vi "BinanceAPI_hmacSHA256.vi"(7 "Key":string, 8 "error In":errorcluster, 11 "String to Encode":string) -> (0 "error Out":errorcluster, 3 "Hash String":string)   [LabVIEW 2022 SP3]
doc: "Calculates the SHA256 HMAC signature"
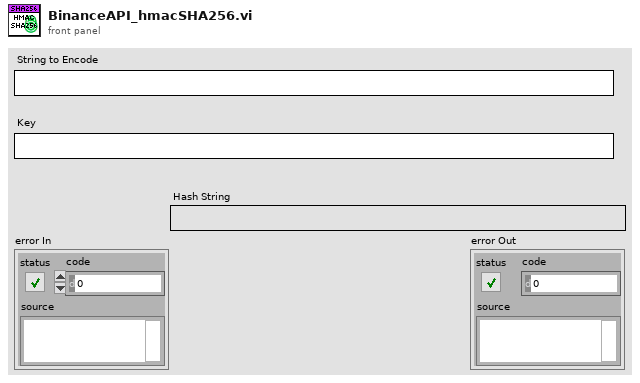
[diagram p1: front panel]
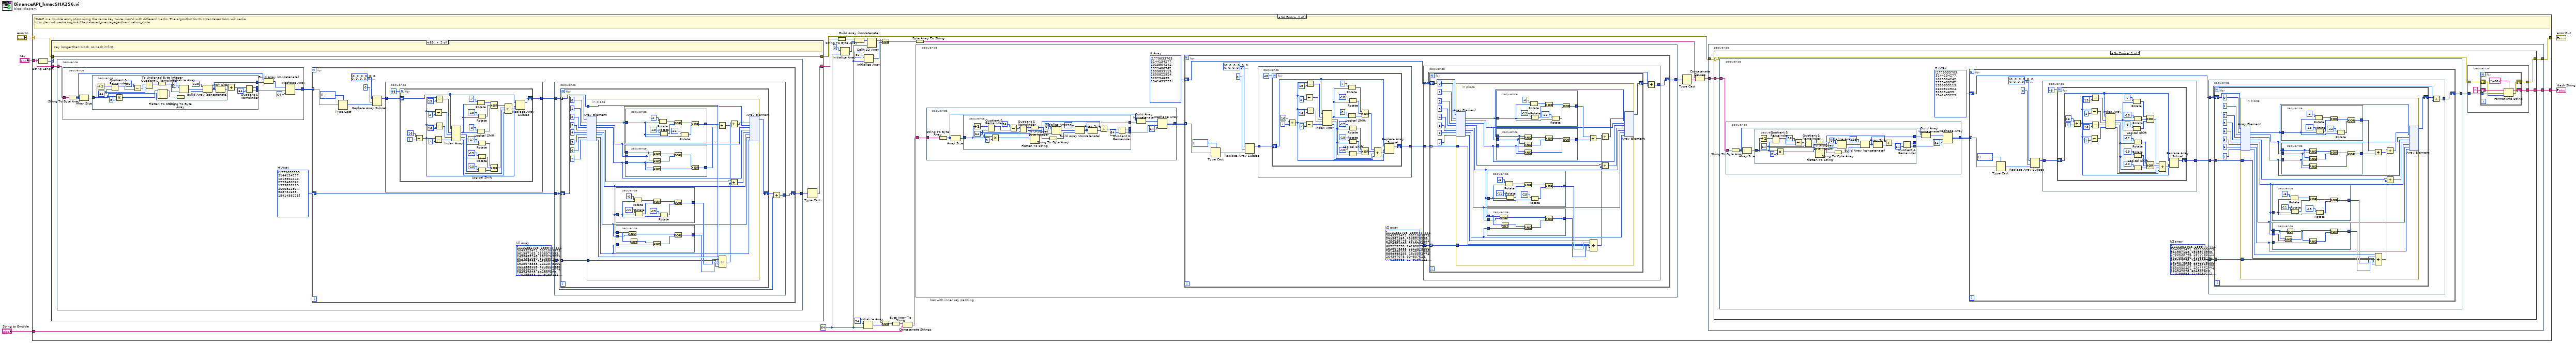
[diagram p0: block diagram]
diagram:
  n1 = case shown="No Error" "error In" {
    selector: "error In" -> [w29 w497]
    tunnel: "Key" -> [w30 _]
    tunnel: "String to Encode" -> [w16 _]
    tunnel: [w13 w497] -> w2
    tunnel: [w12 _] -> w1
    frame No Error {
      w9 = 64 ("dimension size")
      # "has with inner key padding"
      # "HMAC is a double encryption uisng the same key twice, xorr'd with different masks. The algorithm for this was taken from wikipedia \nhttps://en.wikipedia.org/wiki/Hash-based_message_authentication_code"
      n2 = String Length(string=w30) -> (length=w31:i32)
      n3 = case shown="65.." w31 {
        tunnel: w30 -> [w346 w350]
        tunnel: w29 -> [w345 w349]
        tunnel: [w345 w349] -> w11
        tunnel: [w346 w348] -> w28
        frame 0, Default {
        }
        frame 65.. {
          # "Key longer than block, so hash it first."
          n4 = stacked-sequence {
            tunnel: [w353] -> w347
            tunnel: w350 -> [w354]
            frame #0 {
              w351 = u32[] [1779033703, 3144134277, 1013904242, 2773480762, 1359893119, 2600822924, 528734635, 1541459225]  # H Array
              n5 = stacked-sequence {
                tunnel: [w358] -> w352
                tunnel: w354 -> [w355]
                frame #0 {
                  n6 = String To Byte Array(string=w355) -> (unsigned byte array=w359:u8[])
                  n7 = Array Size(array=w359) -> (size(s)=w361:i32)
                  n8 = stacked-sequence {
                    tunnel: [w363] -> _
                    tunnel: [w370] -> w356
                    tunnel: [w365] -> w360
                    tunnel: w361 -> [w379]
                    frame #0 {
                      w368 = i64 64 ("y")
                      n9 = Increment(x=w379) -> (x+1=w378:i32)
                      n10 = Quotient & Remainder(x=w378, y=w368) -> (x-y*floor(x/y)=w377:i64)  [unwired: 1 out]
                      n11 = Multiply(x=w379, y=i64 8) -> (x*y=w383:i64)
                      n12 = Subtract(x=i64 56, y=w377) -> (x-y=w369:i64)
                      n13 = Quotient & Remainder(x=w369, y=w368) -> (x-y*floor(x/y)=w366:i64)  [unwired: 1 out]
                      n14 = To Unsigned Byte Integer(number=w366) -> (unsigned 8bit integer=w380:u8)
                      n15 = Flatten To String(anything=w383) -> (data string=w381:string)  [unwired: 3 in, 2 out]
                      n16 = String To Byte Array(string=w381) -> (unsigned byte array=w382:u8[])
                      n17 = Initialize Array(u8 0, w380) -> (w374:u8[])
                      n18 = Build Array (concatenate)(u8 128, w374, w382) -> (w365:u8[])
                      n19 = Array Size(array=w365) -> (size(s)=w372:i32)
                      n20 = Add(x=w379, y=w372) -> (x+y=w364:i32)
                      n21 = Quotient & Remainder(x=w364, y=u64 64) -> (x-y*floor(x/y)=w363:u64, floor(x/y)=w370:u64)
                    }
                  }
                  n22 = Build Array (concatenate)(w359, w360) -> (w362:u8[])
                  n23 = Reshape Array(w362, w356, 64 ("dimension size")) -> (w358:u8[][])
                }
              }
              n24 = for {
                tunnel: w352 -> [w393] mode=indexing
                shift-right: [w386] -> w353
                shift-left: w351 -> [w387]
                w385 = u32[] [1116352408, 1899447441, 3049323471, 3921009573, 961987163, 1508970993, 2453635748, 2870763221, 3624381080, 310598401, 607225278, 1426881987, 1925078388, 2162078206, 2614888103, 3248222580, 3835390401, 4022224774, 264347078, 604807628, 770255983, 1249150122, 1555081692, 1996064986, 2554220882, 2821834349, 2952996808, 3210313671, 3336571891, 3584528711, 113926993, 338241895, 666307205, 773529912, 1294757372, 1396182291, 1695183700, 1986661051, 2177026350, 2456956037, 2730485921, 2820302411, 3259730800, 3345764771, 3516065817, 3600352804, 4094571909, 275423344, 430227734, 506948616, 659060556, 883997877, 958139571, 1322822218, 1537002063, 1747873779, 1955562222, 2024104815, 2227730452, 2361852424, 2428436474, 2756734187, 3204031479, 3329325298]  # k[] array
                n25 = Type Cast(type=u32[] [], x=w393) -> (*(type *) &x=w391:u32[])
                n26 = Replace Array Subset(array=u32[] [0, 0, 0, 0, 0, 0, 0, 0, 0, 0, 0, 0, 0, 0, 0, 0, 0, 0, 0, 0, 0, 0, 0, 0, 0, 0, 0, 0, 0, 0, 0, 0, 0, 0, 0, 0, 0, 0, 0, 0, 0, 0, 0, 0, 0, 0, 0, 0, 0, 0, 0, 0, 0, 0, 0, 0, 0, 0, 0, 0, 0, 0, 0, 0], new element=w391, index=0) -> (w389:u32[])
                n27 = stacked-sequence {
                  tunnel: [w462] -> w388
                  tunnel: w389 -> [w463]
                  frame #0 {
                    n28 = for {
                      N: 48 -> [_]
                      shift-right: [w467] -> w462
                      shift-left: w463 -> [w490]
                      i -> [w496]
                      n29 = Add(x=16, y=w496) -> (x+y=w465:i32)
                      n30 = Subtract(x=w465, y=2) -> (x-y=w492:i32)
                      n31 = Subtract(x=w465, y=7) -> (x-y=w486:i32)
                      n32 = Subtract(x=w465, y=15) -> (x-y=w494:i32)
                      n33 = Subtract(x=w465, y=16) -> (x-y=w489:i32)
                      n34 = Index Array(array=w490, index #1=w494, index #2=w492, index #3=w489, index #4=w486) -> (element #1=w483:u32, element #2=w476:u32, element #3=w469:u32, element #4=w468:u32)
                      n35 = Rotate(1:w483, 2:i16 -7 ("y")) -> (0:w481:u32)
                      n36 = Logical Shift(y=i16 -3, x=w483) -> (x << y=w479:u32)
                      n37 = Rotate(1:w483, 2:i16 -18 ("y")) -> (0:w480:u32)
                      n38 = Rotate(1:w476, 2:i16 -17 ("y")) -> (0:w472:u32)
                      n39 = Rotate(1:w476, 2:i16 -19 ("y")) -> (0:w473:u32)
                      n40 = Logical Shift(y=i16 -10, x=w476) -> (x << y=w474:u32)
                      n41 = Compound Arithmetic op=XOR(w481, w480, w479) -> (w471:u32)
                      n42 = Compound Arithmetic op=XOR(w472, w473, w474) -> (w470:u32)
                      n43 = Compound Arithmetic op=ADD(w471, w470, w469, w468) -> (w466:u32)
                      n44 = Replace Array Subset(array=w490, new element=w466, index=w465) -> (w467:u32[])
                    }
                  }
                }
                n45 = stacked-sequence {
                  tunnel: [w398] -> w386
                  tunnel: w385 -> [w394]
                  tunnel: w387 -> [w396]
                  tunnel: w388 -> [w395]
                  frame #0 {
                    n46 = for {
                      tunnel: w395 -> [w401] mode=indexing
                      tunnel: w394 -> [w400] mode=indexing
                      shift-right: [w399] -> w397
                      shift-left: w396 -> [w410]
                      n47 = in-place {
                        in-place-border: w401 -> [w425]
                        in-place-border: w400 -> [w424]
                        n48 = in-place-array #1(w410, 0, 1, 2, 3, 4, 5, 6, 7) -> (w414:u32, w415:u32, w416:u32, w418:u32, w419:u32, w420:u32, w421:u32, w428:u32)
                        n49 = stacked-sequence {
                          tunnel: [w444] -> w427
                          tunnel: w419 -> [w439]
                          frame #0 {
                            n50 = Rotate(1:w439, 2:i16 -6 ("y")) -> (0:w440:u32)
                            n51 = Rotate(1:w439, 2:i16 -11 ("y")) -> (0:w441:u32)
                            n52 = Exclusive Or(1:w441, 2:w440) -> (0:w442:u32)
                            n53 = Rotate(1:w439, 2:i16 -25 ("y")) -> (0:w443:u32)
                            n54 = Exclusive Or(1:w443, 2:w442) -> (0:w444:u32)
                          }
                        }
                        n55 = stacked-sequence {
                          tunnel: [w435] -> w426
                          tunnel: w421 -> [w432]
                          tunnel: w420 -> [w429]
                          tunnel: w419 -> [w430]
                          frame #0 {
                            n56 = And(x=w430, y=w429) -> (x .and. y?=w433:u32)
                            n57 = Not(x=w430) -> (.not. x?=w431:u32)
                            n58 = And(x=w431, y=w432) -> (x .and. y?=w434:u32)
                            n59 = Exclusive Or(1:w434, 2:w433) -> (0:w435:u32)
                          }
                        }
                        n60 = stacked-sequence {
                          tunnel: [w461] -> w423
                          tunnel: w414 -> [w456]
                          frame #0 {
                            n61 = Rotate(1:w456, 2:i16 -2 ("y")) -> (0:w457:u32)
                            n62 = Rotate(1:w456, 2:i16 -13 ("y")) -> (0:w458:u32)
                            n63 = Exclusive Or(1:w458, 2:w457) -> (0:w459:u32)
                            n64 = Rotate(1:w456, 2:i16 -22 ("y")) -> (0:w460:u32)
                            n65 = Exclusive Or(1:w460, 2:w459) -> (0:w461:u32)
                          }
                        }
                        n66 = stacked-sequence {
                          tunnel: [w452] -> w422
                          tunnel: w416 -> [w446]
                          tunnel: w415 -> [w445]
                          tunnel: w414 -> [w447]
                          frame #0 {
                            n67 = And(x=w447, y=w445) -> (x .and. y?=w448:u32)
                            n68 = And(x=w447, y=w446) -> (x .and. y?=w449:u32)
                            n69 = And(x=w445, y=w446) -> (x .and. y?=w451:u32)
                            n70 = Exclusive Or(1:w449, 2:w448) -> (0:w450:u32)
                            n71 = Exclusive Or(1:w451, 2:w450) -> (0:w452:u32)
                          }
                        }
                        n72 = Add(x=w423, y=w422) -> (x+y=w412:u32)
                        n73 = Compound Arithmetic op=ADD(w428, w427, w426, w425, w424) -> (w413:u32)
                        n74 = Add(x=w413, y=w412) -> (x+y=w411:u32)
                        n75 = Add(x=w418, y=w413) -> (x+y=w417:u32)
                        n76 = in-place-array #1(w411, w414, w415, w416, w417, w419, w420, w421) -> (w399:u32[])  [unwired: 8 out]
                      }
                    }
                    n77 = Add(x=w397, y=w396) -> (x+y=w398:u32[])
                  }
                }
              }
            }
          }
          n78 = Type Cast(x=w347) -> (*(type *) &x=w348:string)  [unwired: 1 in]
        }
      }
      n79 = String To Byte Array(string=w28) -> (unsigned byte array=w27:u8[])
      n80 = Initialize Array(u8 0 ("element"), w9) -> (w25:u8[])
      n81 = Build Array (concatenate)(w27, w25) -> (w24:u8[])
      n82 = Initialize Array(u8 54, w9) -> (w20:u8[])
      n83 = Initialize Array(u8 92, w9) -> (w21:u8[])
      n84 = Split 1D Array(array=w24, index=w9) -> (first subarray=w19:u8[])  [unwired: 1 out]
      n85 = Exclusive Or(1:w21, 2:w19) -> (0:w18:u8[])
      n86 = Exclusive Or(1:w20, 2:w19) -> (0:w17:u8[])
      n87 = Byte Array To String(unsigned byte array=w17) -> (string=w10:string)
      n88 = Concatenate Strings(w10, w16) -> (w8:string)
      n89 = Byte Array To String(unsigned byte array=w18) -> (string=w15:string)
      n90 = stacked-sequence {
        tunnel: [w201] -> w7
        tunnel: w8 -> [w202]
        frame #0 {
          w199 = u32[] [1779033703, 3144134277, 1013904242, 2773480762, 1359893119, 2600822924, 528734635, 1541459225]  # H Array
          n91 = stacked-sequence {
            tunnel: [w206] -> w200
            tunnel: w202 -> [w203]
            frame #0 {
              n92 = String To Byte Array(string=w203) -> (unsigned byte array=w207:u8[])
              n93 = Array Size(array=w207) -> (size(s)=w209:i32)
              n94 = stacked-sequence {
                tunnel: [w211] -> _
                tunnel: [w218] -> w204
                tunnel: [w213] -> w208
                tunnel: w209 -> [w227]
                frame #0 {
                  w216 = i64 64 ("y")
                  n95 = Increment(x=w227) -> (x+1=w226:i32)
                  n96 = Quotient & Remainder(x=w226, y=w216) -> (x-y*floor(x/y)=w225:i64)  [unwired: 1 out]
                  n97 = Multiply(x=w227, y=i64 8) -> (x*y=w231:i64)
                  n98 = Subtract(x=i64 56, y=w225) -> (x-y=w217:i64)
                  n99 = Quotient & Remainder(x=w217, y=w216) -> (x-y*floor(x/y)=w214:i64)  [unwired: 1 out]
                  n100 = To Unsigned Byte Integer(number=w214) -> (unsigned 8bit integer=w228:u8)
                  n101 = Flatten To String(anything=w231) -> (data string=w229:string)  [unwired: 3 in, 2 out]
                  n102 = String To Byte Array(string=w229) -> (unsigned byte array=w230:u8[])
                  n103 = Initialize Array(u8 0, w228) -> (w222:u8[])
                  n104 = Build Array (concatenate)(u8 128, w222, w230) -> (w213:u8[])
                  n105 = Array Size(array=w213) -> (size(s)=w220:i32)
                  n106 = Add(x=w227, y=w220) -> (x+y=w212:i32)
                  n107 = Quotient & Remainder(x=w212, y=u64 64) -> (x-y*floor(x/y)=w211:u64, floor(x/y)=w218:u64)
                }
              }
              n108 = Build Array (concatenate)(w207, w208) -> (w210:u8[])
              n109 = Reshape Array(w210, w204, 64 ("dimension size")) -> (w206:u8[][])
            }
          }
          n110 = for {
            tunnel: w200 -> [w241] mode=indexing
            shift-right: [w234] -> w201
            shift-left: w199 -> [w235]
            w233 = u32[] [1116352408, 1899447441, 3049323471, 3921009573, 961987163, 1508970993, 2453635748, 2870763221, 3624381080, 310598401, 607225278, 1426881987, 1925078388, 2162078206, 2614888103, 3248222580, 3835390401, 4022224774, 264347078, 604807628, 770255983, 1249150122, 1555081692, 1996064986, 2554220882, 2821834349, 2952996808, 3210313671, 3336571891, 3584528711, 113926993, 338241895, 666307205, 773529912, 1294757372, 1396182291, 1695183700, 1986661051, 2177026350, 2456956037, 2730485921, 2820302411, 3259730800, 3345764771, 3516065817, 3600352804, 4094571909, 275423344, 430227734, 506948616, 659060556, 883997877, 958139571, 1322822218, 1537002063, 1747873779, 1955562222, 2024104815, 2227730452, 2361852424, 2428436474, 2756734187, 3204031479, 3329325298]  # k[] array
            n111 = Type Cast(type=u32[] [], x=w241) -> (*(type *) &x=w239:u32[])
            n112 = Replace Array Subset(array=u32[] [0, 0, 0, 0, 0, 0, 0, 0, 0, 0, 0, 0, 0, 0, 0, 0, 0, 0, 0, 0, 0, 0, 0, 0, 0, 0, 0, 0, 0, 0, 0, 0, 0, 0, 0, 0, 0, 0, 0, 0, 0, 0, 0, 0, 0, 0, 0, 0, 0, 0, 0, 0, 0, 0, 0, 0, 0, 0, 0, 0, 0, 0, 0, 0], new element=w239, index=0) -> (w237:u32[])
            n113 = stacked-sequence {
              tunnel: [w310] -> w236
              tunnel: w237 -> [w311]
              frame #0 {
                n114 = for {
                  N: 48 -> [_]
                  shift-right: [w315] -> w310
                  shift-left: w311 -> [w338]
                  i -> [w344]
                  n115 = Add(x=16, y=w344) -> (x+y=w313:i32)
                  n116 = Subtract(x=w313, y=2) -> (x-y=w340:i32)
                  n117 = Subtract(x=w313, y=7) -> (x-y=w334:i32)
                  n118 = Subtract(x=w313, y=15) -> (x-y=w342:i32)
                  n119 = Subtract(x=w313, y=16) -> (x-y=w337:i32)
                  n120 = Index Array(array=w338, index #1=w342, index #2=w340, index #3=w337, index #4=w334) -> (element #1=w331:u32, element #2=w324:u32, element #3=w317:u32, element #4=w316:u32)
                  n121 = Rotate(1:w331, 2:i16 -7 ("y")) -> (0:w329:u32)
                  n122 = Logical Shift(y=i16 -3, x=w331) -> (x << y=w327:u32)
                  n123 = Rotate(1:w331, 2:i16 -18 ("y")) -> (0:w328:u32)
                  n124 = Rotate(1:w324, 2:i16 -17 ("y")) -> (0:w320:u32)
                  n125 = Rotate(1:w324, 2:i16 -19 ("y")) -> (0:w321:u32)
                  n126 = Logical Shift(y=i16 -10, x=w324) -> (x << y=w322:u32)
                  n127 = Compound Arithmetic op=XOR(w329, w328, w327) -> (w319:u32)
                  n128 = Compound Arithmetic op=XOR(w320, w321, w322) -> (w318:u32)
                  n129 = Compound Arithmetic op=ADD(w319, w318, w317, w316) -> (w314:u32)
                  n130 = Replace Array Subset(array=w338, new element=w314, index=w313) -> (w315:u32[])
                }
              }
            }
            n131 = stacked-sequence {
              tunnel: [w246] -> w234
              tunnel: w233 -> [w242]
              tunnel: w235 -> [w244]
              tunnel: w236 -> [w243]
              frame #0 {
                n132 = for {
                  tunnel: w243 -> [w249] mode=indexing
                  tunnel: w242 -> [w248] mode=indexing
                  shift-right: [w247] -> w245
                  shift-left: w244 -> [w258]
                  n133 = in-place {
                    in-place-border: w249 -> [w273]
                    in-place-border: w248 -> [w272]
                    n134 = in-place-array #2(w258, 0, 1, 2, 3, 4, 5, 6, 7) -> (w262:u32, w263:u32, w264:u32, w266:u32, w267:u32, w268:u32, w269:u32, w276:u32)
                    n135 = stacked-sequence {
                      tunnel: [w292] -> w275
                      tunnel: w267 -> [w287]
                      frame #0 {
                        n136 = Rotate(1:w287, 2:i16 -6 ("y")) -> (0:w288:u32)
                        n137 = Rotate(1:w287, 2:i16 -11 ("y")) -> (0:w289:u32)
                        n138 = Exclusive Or(1:w289, 2:w288) -> (0:w290:u32)
                        n139 = Rotate(1:w287, 2:i16 -25 ("y")) -> (0:w291:u32)
                        n140 = Exclusive Or(1:w291, 2:w290) -> (0:w292:u32)
                      }
                    }
                    n141 = stacked-sequence {
                      tunnel: [w283] -> w274
                      tunnel: w269 -> [w280]
                      tunnel: w268 -> [w277]
                      tunnel: w267 -> [w278]
                      frame #0 {
                        n142 = And(x=w278, y=w277) -> (x .and. y?=w281:u32)
                        n143 = Not(x=w278) -> (.not. x?=w279:u32)
                        n144 = And(x=w279, y=w280) -> (x .and. y?=w282:u32)
                        n145 = Exclusive Or(1:w282, 2:w281) -> (0:w283:u32)
                      }
                    }
                    n146 = stacked-sequence {
                      tunnel: [w309] -> w271
                      tunnel: w262 -> [w304]
                      frame #0 {
                        n147 = Rotate(1:w304, 2:i16 -2 ("y")) -> (0:w305:u32)
                        n148 = Rotate(1:w304, 2:i16 -13 ("y")) -> (0:w306:u32)
                        n149 = Exclusive Or(1:w306, 2:w305) -> (0:w307:u32)
                        n150 = Rotate(1:w304, 2:i16 -22 ("y")) -> (0:w308:u32)
                        n151 = Exclusive Or(1:w308, 2:w307) -> (0:w309:u32)
                      }
                    }
                    n152 = stacked-sequence {
                      tunnel: [w300] -> w270
                      tunnel: w264 -> [w294]
                      tunnel: w263 -> [w293]
                      tunnel: w262 -> [w295]
                      frame #0 {
                        n153 = And(x=w295, y=w293) -> (x .and. y?=w296:u32)
                        n154 = And(x=w295, y=w294) -> (x .and. y?=w297:u32)
                        n155 = And(x=w293, y=w294) -> (x .and. y?=w299:u32)
                        n156 = Exclusive Or(1:w297, 2:w296) -> (0:w298:u32)
                        n157 = Exclusive Or(1:w299, 2:w298) -> (0:w300:u32)
                      }
                    }
                    n158 = Add(x=w271, y=w270) -> (x+y=w260:u32)
                    n159 = Compound Arithmetic op=ADD(w276, w275, w274, w273, w272) -> (w261:u32)
                    n160 = Add(x=w261, y=w260) -> (x+y=w259:u32)
                    n161 = Add(x=w266, y=w261) -> (x+y=w265:u32)
                    n162 = in-place-array #2(w259, w262, w263, w264, w265, w267, w268, w269) -> (w247:u32[])  [unwired: 8 out]
                  }
                }
                n163 = Add(x=w245, y=w244) -> (x+y=w246:u32[])
              }
            }
          }
        }
      }
      n164 = Type Cast(x=w7) -> (*(type *) &x=w6:string)  [unwired: 1 in]
      n165 = Concatenate Strings(w15, w6) -> (w14:string)
      n166 = stacked-sequence {
        tunnel: [w34] -> w13
        tunnel: [w33] -> w12
        tunnel: w11 -> [w35]
        tunnel: w14 -> [w32]
        frame #0 {
          n167 = case shown="No Error" w35 {
            selector: w35 -> [w36 w198]
            tunnel: w32 -> [w40 _]
            tunnel: [w38 _] -> w33
            tunnel: [w37 w198] -> w34
            frame No Error {
              n168 = stacked-sequence {
                tunnel: [w54] -> w39
                tunnel: w40 -> [w55]
                frame #0 {
                  w52 = u32[] [1779033703, 3144134277, 1013904242, 2773480762, 1359893119, 2600822924, 528734635, 1541459225]  # H Array
                  n169 = stacked-sequence {
                    tunnel: [w59] -> w53
                    tunnel: w55 -> [w56]
                    frame #0 {
                      n170 = String To Byte Array(string=w56) -> (unsigned byte array=w60:u8[])
                      n171 = Array Size(array=w60) -> (size(s)=w62:i32)
                      n172 = stacked-sequence {
                        tunnel: [w64] -> _
                        tunnel: [w71] -> w57
                        tunnel: [w66] -> w61
                        tunnel: w62 -> [w80]
                        frame #0 {
                          w69 = i64 64 ("y")
                          n173 = Increment(x=w80) -> (x+1=w79:i32)
                          n174 = Quotient & Remainder(x=w79, y=w69) -> (x-y*floor(x/y)=w78:i64)  [unwired: 1 out]
                          n175 = Multiply(x=w80, y=i64 8) -> (x*y=w84:i64)
                          n176 = Subtract(x=i64 56, y=w78) -> (x-y=w70:i64)
                          n177 = Quotient & Remainder(x=w70, y=w69) -> (x-y*floor(x/y)=w67:i64)  [unwired: 1 out]
                          n178 = To Unsigned Byte Integer(number=w67) -> (unsigned 8bit integer=w81:u8)
                          n179 = Flatten To String(anything=w84) -> (data string=w82:string)  [unwired: 3 in, 2 out]
                          n180 = String To Byte Array(string=w82) -> (unsigned byte array=w83:u8[])
                          n181 = Initialize Array(u8 0, w81) -> (w75:u8[])
                          n182 = Build Array (concatenate)(u8 128, w75, w83) -> (w66:u8[])
                          n183 = Array Size(array=w66) -> (size(s)=w73:i32)
                          n184 = Add(x=w80, y=w73) -> (x+y=w65:i32)
                          n185 = Quotient & Remainder(x=w65, y=u64 64) -> (x-y*floor(x/y)=w64:u64, floor(x/y)=w71:u64)
                        }
                      }
                      n186 = Build Array (concatenate)(w60, w61) -> (w63:u8[])
                      n187 = Reshape Array(w63, w57, 64 ("dimension size")) -> (w59:u8[][])
                    }
                  }
                  n188 = for {
                    tunnel: w53 -> [w94] mode=indexing
                    shift-right: [w87] -> w54
                    shift-left: w52 -> [w88]
                    w86 = u32[] [1116352408, 1899447441, 3049323471, 3921009573, 961987163, 1508970993, 2453635748, 2870763221, 3624381080, 310598401, 607225278, 1426881987, 1925078388, 2162078206, 2614888103, 3248222580, 3835390401, 4022224774, 264347078, 604807628, 770255983, 1249150122, 1555081692, 1996064986, 2554220882, 2821834349, 2952996808, 3210313671, 3336571891, 3584528711, 113926993, 338241895, 666307205, 773529912, 1294757372, 1396182291, 1695183700, 1986661051, 2177026350, 2456956037, 2730485921, 2820302411, 3259730800, 3345764771, 3516065817, 3600352804, 4094571909, 275423344, 430227734, 506948616, 659060556, 883997877, 958139571, 1322822218, 1537002063, 1747873779, 1955562222, 2024104815, 2227730452, 2361852424, 2428436474, 2756734187, 3204031479, 3329325298]  # k[] array
                    n189 = Type Cast(type=u32[] [], x=w94) -> (*(type *) &x=w92:u32[])
                    n190 = Replace Array Subset(array=u32[] [0, 0, 0, 0, 0, 0, 0, 0, 0, 0, 0, 0, 0, 0, 0, 0, 0, 0, 0, 0, 0, 0, 0, 0, 0, 0, 0, 0, 0, 0, 0, 0, 0, 0, 0, 0, 0, 0, 0, 0, 0, 0, 0, 0, 0, 0, 0, 0, 0, 0, 0, 0, 0, 0, 0, 0, 0, 0, 0, 0, 0, 0, 0, 0], new element=w92, index=0) -> (w90:u32[])
                    n191 = stacked-sequence {
                      tunnel: [w163] -> w89
                      tunnel: w90 -> [w164]
                      frame #0 {
                        n192 = for {
                          N: 48 -> [_]
                          shift-right: [w168] -> w163
                          shift-left: w164 -> [w191]
                          i -> [w197]
                          n193 = Add(x=16, y=w197) -> (x+y=w166:i32)
                          n194 = Subtract(x=w166, y=2) -> (x-y=w193:i32)
                          n195 = Subtract(x=w166, y=7) -> (x-y=w187:i32)
                          n196 = Subtract(x=w166, y=15) -> (x-y=w195:i32)
                          n197 = Subtract(x=w166, y=16) -> (x-y=w190:i32)
                          n198 = Index Array(array=w191, index #1=w195, index #2=w193, index #3=w190, index #4=w187) -> (element #1=w184:u32, element #2=w177:u32, element #3=w170:u32, element #4=w169:u32)
                          n199 = Rotate(1:w184, 2:i16 -7 ("y")) -> (0:w182:u32)
                          n200 = Logical Shift(y=i16 -3, x=w184) -> (x << y=w180:u32)
                          n201 = Rotate(1:w184, 2:i16 -18 ("y")) -> (0:w181:u32)
                          n202 = Rotate(1:w177, 2:i16 -17 ("y")) -> (0:w173:u32)
                          n203 = Rotate(1:w177, 2:i16 -19 ("y")) -> (0:w174:u32)
                          n204 = Logical Shift(y=i16 -10, x=w177) -> (x << y=w175:u32)
                          n205 = Compound Arithmetic op=XOR(w182, w181, w180) -> (w172:u32)
                          n206 = Compound Arithmetic op=XOR(w173, w174, w175) -> (w171:u32)
                          n207 = Compound Arithmetic op=ADD(w172, w171, w170, w169) -> (w167:u32)
                          n208 = Replace Array Subset(array=w191, new element=w167, index=w166) -> (w168:u32[])
                        }
                      }
                    }
                    n209 = stacked-sequence {
                      tunnel: [w99] -> w87
                      tunnel: w86 -> [w95]
                      tunnel: w88 -> [w97]
                      tunnel: w89 -> [w96]
                      frame #0 {
                        n210 = for {
                          tunnel: w96 -> [w102] mode=indexing
                          tunnel: w95 -> [w101] mode=indexing
                          shift-right: [w100] -> w98
                          shift-left: w97 -> [w111]
                          n211 = in-place {
                            in-place-border: w102 -> [w126]
                            in-place-border: w101 -> [w125]
                            n212 = in-place-array #3(w111, 0, 1, 2, 3, 4, 5, 6, 7) -> (w115:u32, w116:u32, w117:u32, w119:u32, w120:u32, w121:u32, w122:u32, w129:u32)
                            n213 = stacked-sequence {
                              tunnel: [w153] -> w128
                              tunnel: w120 -> [w148]
                              frame #0 {
                                n214 = Rotate(1:w148, 2:i16 -6 ("y")) -> (0:w149:u32)
                                n215 = Rotate(1:w148, 2:i16 -11 ("y")) -> (0:w150:u32)
                                n216 = Exclusive Or(1:w150, 2:w149) -> (0:w151:u32)
                                n217 = Rotate(1:w148, 2:i16 -25 ("y")) -> (0:w152:u32)
                                n218 = Exclusive Or(1:w152, 2:w151) -> (0:w153:u32)
                              }
                            }
                            n219 = stacked-sequence {
                              tunnel: [w136] -> w127
                              tunnel: w122 -> [w133]
                              tunnel: w121 -> [w130]
                              tunnel: w120 -> [w131]
                              frame #0 {
                                n220 = And(x=w131, y=w130) -> (x .and. y?=w134:u32)
                                n221 = Not(x=w131) -> (.not. x?=w132:u32)
                                n222 = And(x=w132, y=w133) -> (x .and. y?=w135:u32)
                                n223 = Exclusive Or(1:w135, 2:w134) -> (0:w136:u32)
                              }
                            }
                            n224 = stacked-sequence {
                              tunnel: [w162] -> w124
                              tunnel: w115 -> [w157]
                              frame #0 {
                                n225 = Rotate(1:w157, 2:i16 -2 ("y")) -> (0:w158:u32)
                                n226 = Rotate(1:w157, 2:i16 -13 ("y")) -> (0:w159:u32)
                                n227 = Exclusive Or(1:w159, 2:w158) -> (0:w160:u32)
                                n228 = Rotate(1:w157, 2:i16 -22 ("y")) -> (0:w161:u32)
                                n229 = Exclusive Or(1:w161, 2:w160) -> (0:w162:u32)
                              }
                            }
                            n230 = stacked-sequence {
                              tunnel: [w144] -> w123
                              tunnel: w117 -> [w138]
                              tunnel: w116 -> [w137]
                              tunnel: w115 -> [w139]
                              frame #0 {
                                n231 = And(x=w139, y=w137) -> (x .and. y?=w140:u32)
                                n232 = And(x=w139, y=w138) -> (x .and. y?=w141:u32)
                                n233 = And(x=w137, y=w138) -> (x .and. y?=w143:u32)
                                n234 = Exclusive Or(1:w141, 2:w140) -> (0:w142:u32)
                                n235 = Exclusive Or(1:w143, 2:w142) -> (0:w144:u32)
                              }
                            }
                            n236 = Add(x=w124, y=w123) -> (x+y=w113:u32)
                            n237 = Compound Arithmetic op=ADD(w129, w128, w127, w126, w125) -> (w114:u32)
                            n238 = Add(x=w114, y=w113) -> (x+y=w112:u32)
                            n239 = Add(x=w119, y=w114) -> (x+y=w118:u32)
                            n240 = in-place-array #3(w112, w115, w116, w117, w118, w120, w121, w122) -> (w100:u32[])  [unwired: 8 out]
                          }
                        }
                        n241 = Add(x=w98, y=w97) -> (x+y=w99:u32[])
                      }
                    }
                  }
                }
              }
              n242 = stacked-sequence {
                tunnel: [w42] -> w37
                tunnel: [w43] -> w38
                tunnel: w36 -> [w41]
                tunnel: w39 -> [w45]
                frame #0 {
                  n243 = for {
                    tunnel: w45 -> [w51] mode=indexing
                    shift-right: [w50] -> w43
                    shift-left: "" -> [w49]
                    shift-right: [w47] -> w42
                    shift-left: w41 -> [w46]
                    n244 = Format Into String(format string="%08x", initial string=w49, error in=w46, w51) -> (resulting string=w50:string, error out=w47:errorcluster)
                  }
                }
              }
            }
            frame Error {
            }
          }
        }
      }
    }
    frame Error {
    }
  }
  "Hash String" <- w1
  "error Out" <- w2
